vi "Read Power Measurement.vi"(8 "error in (no error)":errorcluster, 10 "Power Measurement Type (0: DC Power)":u16(ring) items=["DC Power", "Real Power", "Apparent Power", "Reactive Power", "Power Factor", "Total Power"], 11 "VISA resource name":refnum<visa-resource-name>) -> (0 "error out":errorcluster, 2 "Power Measurement":dbl, 3 "VISA resource name out":refnum<visa-resource-name>)   [LabVIEW 2013, in "California Instruments iX Series.lvlib"]
doc: "Reads the power measurement based on the measurement type chosen."
uses:
  California Instruments iX Series.lvlib
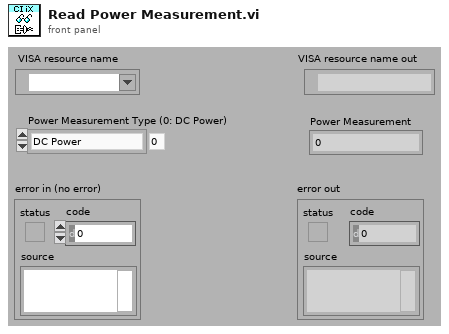
[diagram p1: front panel]
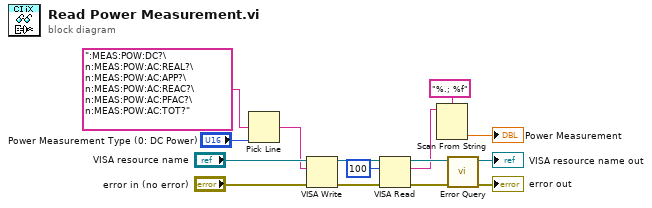
[diagram p0: block diagram]
diagram:
  n1 = Pick Line(multi-line string=":MEAS:POW:DC?\n:MEAS:POW:AC:REAL?\n:MEAS:POW:AC:APP?\n:MEAS:POW:AC:REAC?\n:MEAS:POW:AC:PFAC?\n:MEAS:POW:AC:TOT?", line index="Power Measurement Type (0: DC Power)") -> (output string=w4:string)  [unwired: 1 in]
  n2 = VISA Write(VISA resource name="VISA resource name", write buffer=w4, error in (no error)="error in (no error)") -> (VISA resource name out=w11:refnum<visa-resource-name>, error out=w10:errorcluster)  [unwired: 1 out]
  n3 = VISA Read(VISA resource name=w11, byte count=u32 100, error in (no error)=w10) -> (VISA resource name out=w9:refnum<visa-resource-name>, read buffer=w3:string, error out=w8:errorcluster)  [unwired: 1 out]
  n4 = Scan From String(format string="%.; %f", input string=w3) -> (output 1=→"Power Measurement":dbl)  [unwired: 3 in, 3 out]
  n5 = call "Error Query.vi"("error in (no error)"=w8, "VISA resource name"=w9) -> ("error out"=→"error out":errorcluster, "VISA resource name out"=→"VISA resource name out":refnum<visa-resource-name>)  [unwired: 6 in, 2 out]
